vi "Save Data Functional Global.vi"(6 "Input Parameters":T1={"Points Per A-Scan"=0, "A-Scans per B-Scan"=0, "Voltage Range"=4.0, "Card Resolution (bits)"=16}, 7 "States":T2=enum."Initialize", 8 "error in (no error)":errorcluster, 9 "Folder":path, 10 "U16 Array":u16[](array[numeric]), 11 "Data Format":T3) -> (0 "error out":errorcluster, 3 "Saving Queue Out":refnum<queue>, 4 "# elements in queue":i32, 5 "Time Out":bool)   [LabVIEW 2014]
doc: "Functional global for saving OCT data. The data can either be 1 channel, 2 channel interleaved (ex. ATS 9462), or 2 channels appended (ATS 660). A state exists where the folder and files are created. Once this is complete, data can be enqueued to the VI."
uses:
  Type Defs/OCT DAQ Channel Data Type.ctl
  Saving Data States.ctl
  Type Defs/OCT Imaging Parameters Cluster.ctl
panel:
  out "Numeric":i32
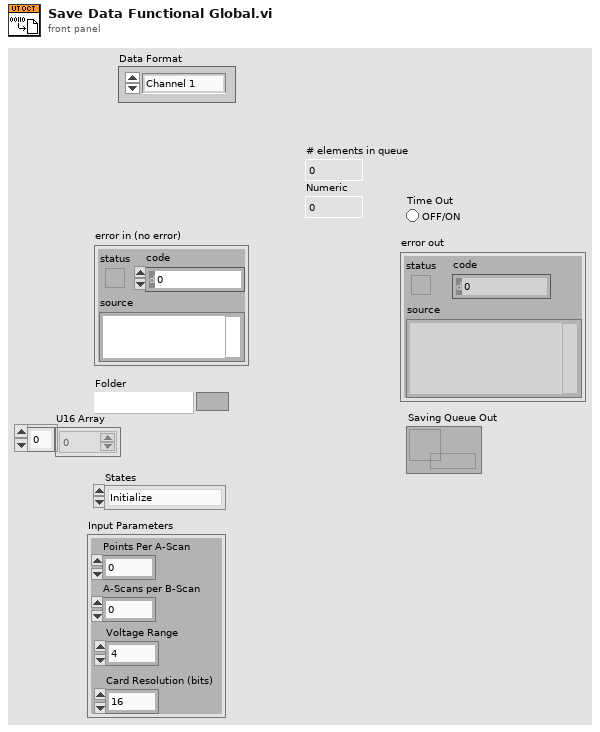
[diagram p1: front panel]
types:
  T1 = typedef "OCT Imaging Parameters Cluster.ctl" = cluster{"Points Per A-Scan":i32, "A-Scans per B-Scan":i32, "Voltage Range":sgl, "Card Resolution (bits)":u16}
  T2 = typedef "Saving Data States.ctl" = enum16{"Get Queue Size", "Get Queue", "Get Timeout", "Flush Queue", "Close Files", "Create Files", "Do Nothing", "Initialize", "Enqueue Data", "Save Data", "Shutdown"}
  T3 = typedef "OCT DAQ Channel Data Type.ctl" = enum16{"Channel 1", "Channel 2", "Channel 1 and 2"}
  T4 = enum16{"open", "replace", "create", "open or create", "replace or create", "replace or create with confirmation"}
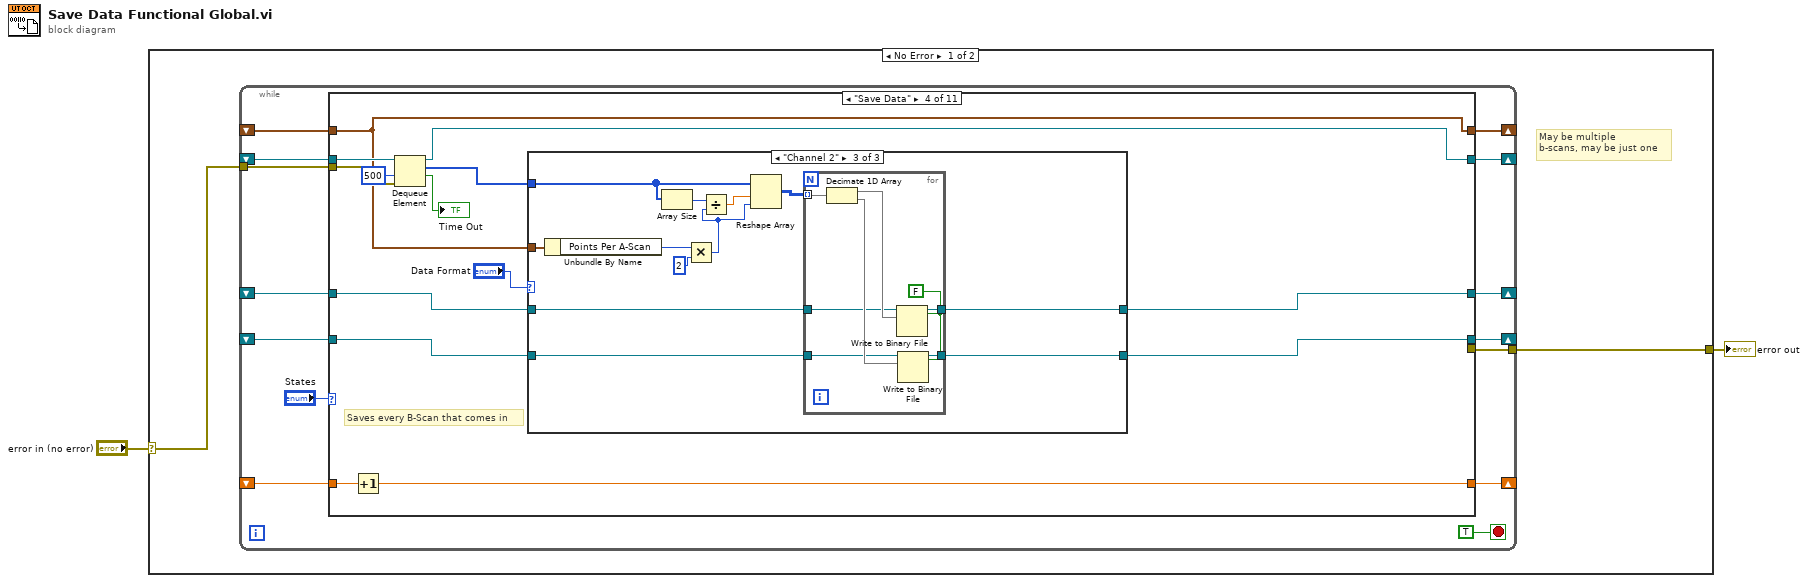
[diagram p0: block diagram]
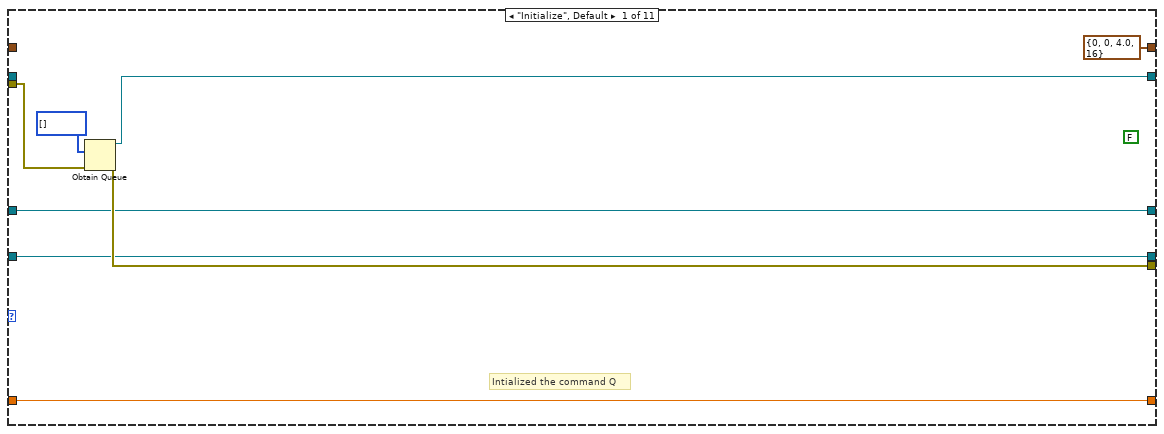
[diagram p2: hidden frame]
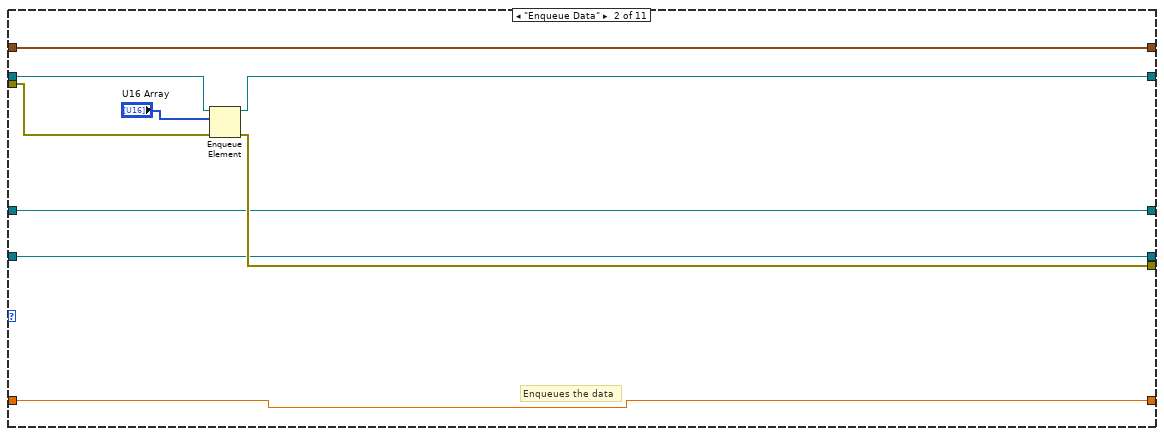
[diagram p3: hidden frame]
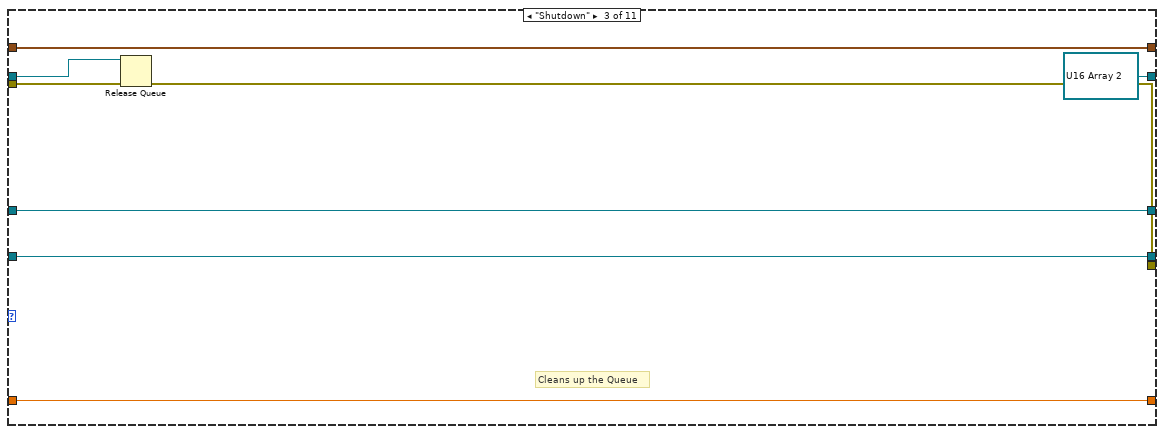
[diagram p4: hidden frame]
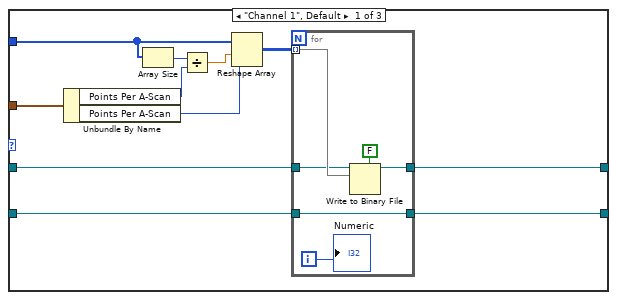
[diagram p5: hidden frame]
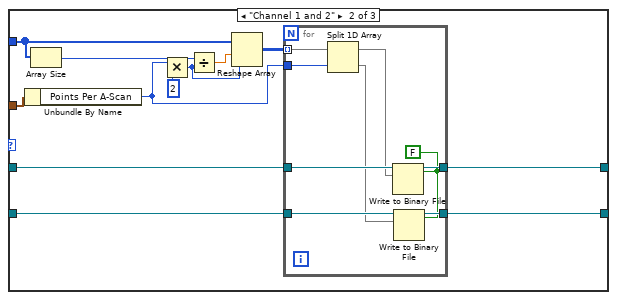
[diagram p6: hidden frame]
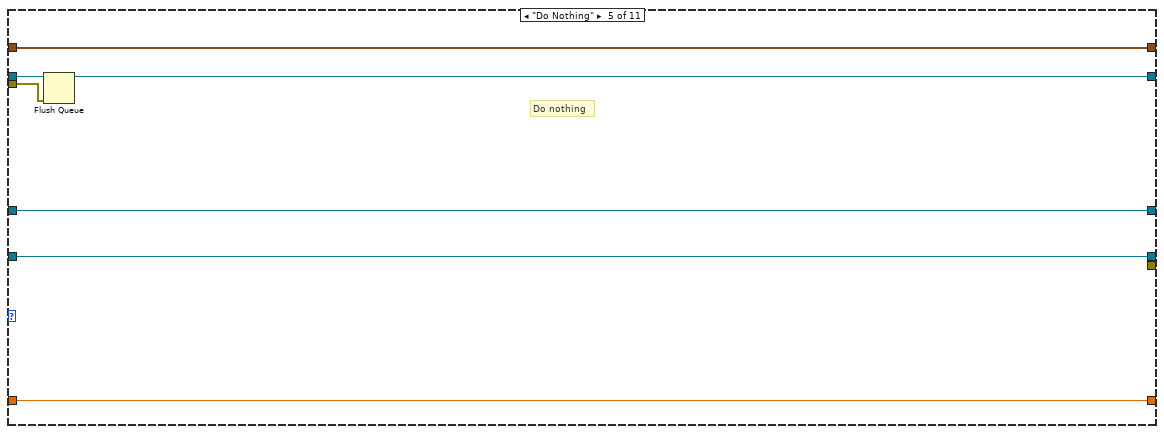
[diagram p7: hidden frame]
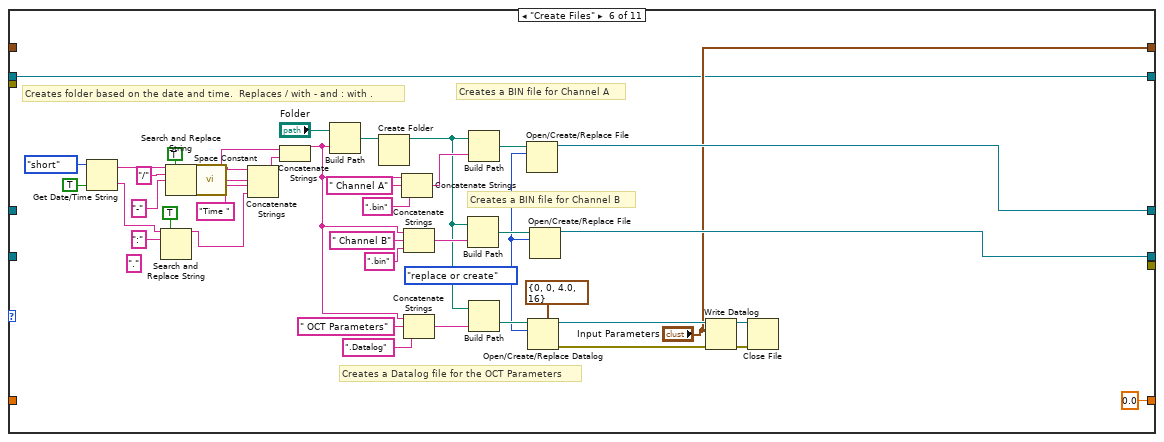
[diagram p8: hidden frame]
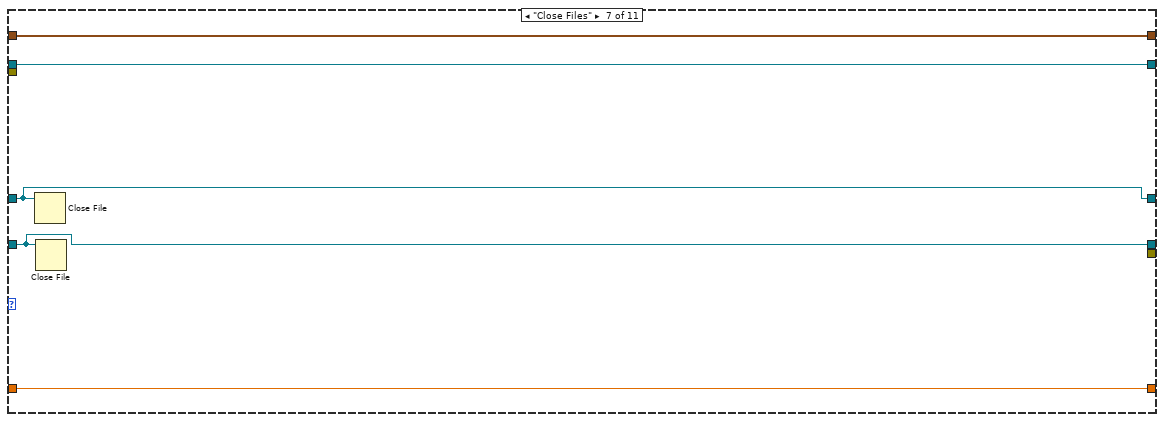
[diagram p9: hidden frame]
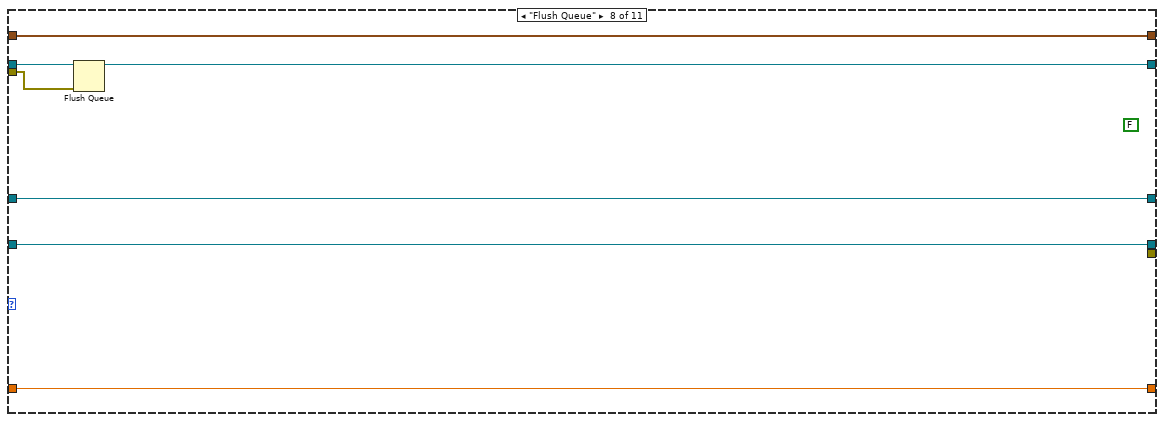
[diagram p10: hidden frame]
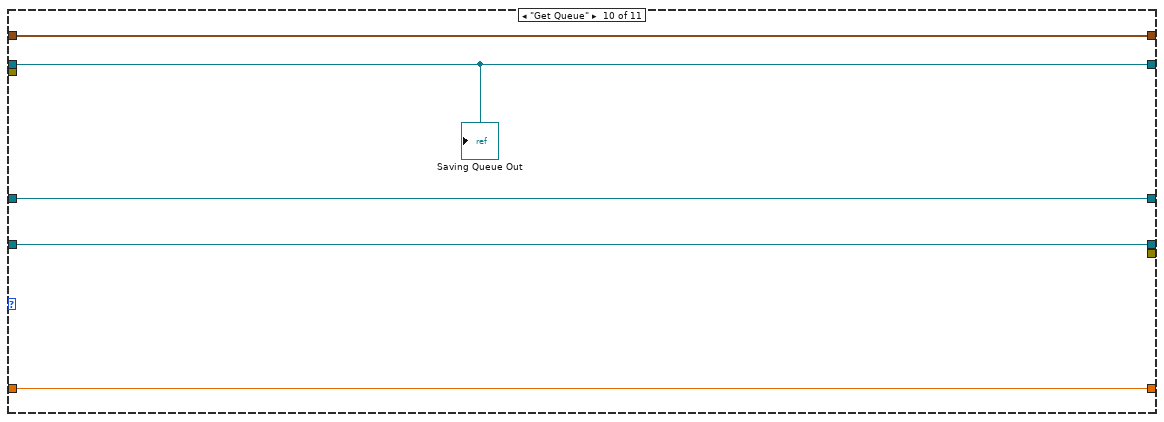
[diagram p12: hidden frame]
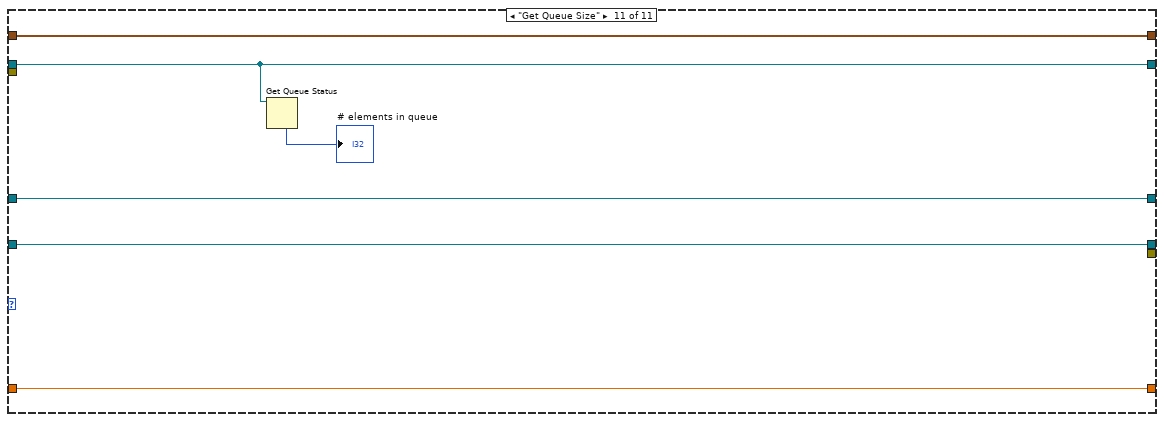
[diagram p13: hidden frame]
diagram:
  n1 = case shown="No Error" "error in (no error)" {
    selector: "error in (no error)" -> [w4 w192]
    tunnel: [w3 w192] -> w1
    frame No Error {
      # "May be multiple\nb-scans, may be just one"
      n2 = while {
        shift-right: [w12] -> _
        shift-left: _ -> [w16]
        tunnel: w4 -> [w17]
        tunnel: [w15] -> w3
        shift-right: [w14] -> _
        shift-left: _ -> [w13]
        shift-right: [w10] -> _
        shift-left: _ -> [w9]
        shift-right: [w8] -> _
        shift-left: _ -> [w7]
        shift-right: [w5] -> _
        shift-left: _ -> [w6]
        stop <- TRUE stop-if-true
        n3 = case shown="\"Save Data\"" "States" {
          tunnel: [w25 w34 refnum<queue> refnum ("queue out") w56 w117 w124 w165 w170 w177 w185 w188] -> w12
          tunnel: w17 -> [w26 w33 w41 w55 w118 _ _ w171 _ _ _]
          tunnel: w16 -> [_ w35 w43 w57 w119 w124 w165 w172 w177 w185 w188]
          tunnel: [w24 w32 w40 _ _ _ _ _ _ _ _] -> w15
          tunnel: [T1 {"Points Per A-Scan"=0, "A-Scans per B-Scan"=0, "Voltage Range"=4.0, "Card Resolution (bits)"=16} ("Input Parameters") w31 w42 w54 w122 "Input Parameters" w166 w173 w178 w184 w191] -> w14
          tunnel: w13 -> [_ w31 w42 w54 w122 _ w166 w173 w178 w184 w191]
          tunnel: [w22 w30 w39 w51 w121 w145 w167 w175 w180 w183 w190] -> w10
          tunnel: w9 -> [w22 w30 w39 w50 w121 _ w167 w175 w180 w183 w190]
          tunnel: [w21 w29 w38 w49 w120 w138 w168 w174 w179 w182 w189] -> w8
          tunnel: w7 -> [w21 w29 w38 w48 w120 _ w168 w174 w179 w182 w189]
          tunnel: w6 -> [w19 w27 w36 w45 w116 _ w164 w169 w176 w181 w186]
          tunnel: [w19 w27 w36 w44 w116 0.0 w164 w169 w176 w181 w186] -> w5
          frame "Initialize", Default {
            (unwired) FALSE ("timed out?")
            # "Intialized the command Q"
            n4 = Obtain Queue(element data type=u16[] [] ("U16 Array 2"), error in (no error)=w26) -> (queue out=w25:refnum<queue>, error out=w24:errorcluster)  [unwired: 3 in, 1 out]
          }
          frame "Enqueue Data" {
            # "Enqueues the data"
            n5 = Enqueue Element(queue=w35, element="U16 Array", error in (no error)=w33) -> (queue out=w34:refnum<queue>, error out=w32:errorcluster)  [unwired: 1 in, 1 out]
          }
          frame "Shutdown" {
            # "Cleans up the Queue"
            n6 = Release Queue(queue=w43, error in (no error)=w41) -> (error out=w40:errorcluster)  [unwired: 1 in, 2 out]
          }
          frame "Save Data" {
            # "Saves every B-Scan that comes in"
            n7 = Increment(x=w45) -> (x+1=w44:dbl)
            n8 = Dequeue Element(queue=w57, timeout in ms (-1)=500, error in (no error)=w55) -> (queue out=w56:refnum<queue>, element=w46:u16[], timed out?=→"Time Out":bool)  [unwired: 1 out]
            n9 = case shown="\"Channel 2\"" "Data Format" {
              tunnel: w46 -> [w65 w84 w105]
              tunnel: w54 -> [w66 w85 w106]
              tunnel: [w63 w81 w103] -> w51
              tunnel: w50 -> [w58 w78 w102]
              tunnel: w48 -> [w62 w79 w101]
              tunnel: [w61 w80 w100] -> w49
              frame "Channel 1", Default {
                n10 = Unbundle By Name(w66) -> ("Points Per A-Scan"=w68:i32, "Points Per A-Scan"=w59:i32)
                n11 = Array Size(array=w65) -> (size(s)=w67:i32)
                n12 = Divide(x=w67, y=w68) -> (x/y=w60:dbl)
                n13 = Reshape Array(w65, w60, w59) -> (w64:u16[][])
                n14 = for {
                  tunnel: w64 -> [w73] mode=indexing
                  tunnel: [w74] -> w63
                  tunnel: w62 -> [w71]
                  tunnel: [w71] -> w61
                  tunnel: w58 -> [w70]
                  i -> [w69]
                  n15 = Write to Binary File(file (use dialog)=w70, data=w73, 5:FALSE ("prepend array or string size? (T)")) -> (refnum out=w74:refnum<file>)  [unwired: 3 in, 2 out]
                  "Numeric" <- w69
                }
              }
              frame "Channel 1 and 2" {
                n16 = Unbundle By Name(w85) -> ("Points Per A-Scan"=w75:i32)
                n17 = Array Size(array=w84) -> (size(s)=w86:i32)
                n18 = Multiply(x=w75, y=2) -> (x*y=w76:i32)
                n19 = Divide(x=w86, y=w76) -> (x/y=w77:dbl)
                n20 = Reshape Array(w84, w77, w76) -> (w82:u16[][])
                n21 = for {
                  tunnel: w82 -> [w95] mode=indexing
                  tunnel: w75 -> [w94]
                  tunnel: [w93] -> w81
                  tunnel: [w92] -> w80
                  tunnel: w79 -> [w91]
                  tunnel: w78 -> [w90]
                  w87 = FALSE ("prepend array or string size? (T)")
                  n22 = Split 1D Array(array=w95, index=w94) -> (first subarray=w89:u16[], second subarray=w88:u16[])
                  n23 = Write to Binary File(file (use dialog)=w90, data=w89, 5:w87) -> (refnum out=w93:refnum<file>)  [unwired: 3 in, 2 out]
                  n24 = Write to Binary File(file (use dialog)=w91, data=w88, 5:w87) -> (refnum out=w92:refnum<file>)  [unwired: 3 in, 2 out]
                }
              }
              frame "Channel 2" {
                n25 = Unbundle By Name(w106) -> ("Points Per A-Scan"=w98:i32)
                n26 = Array Size(array=w105) -> (size(s)=w107:i32)
                n27 = Multiply(x=w98, y=2) -> (x*y=w96:i32)
                n28 = Divide(x=w107, y=w96) -> (x/y=w99:dbl)
                n29 = Reshape Array(w105, w99, w96) -> (w104:u16[][])
                n30 = for {
                  tunnel: w104 -> [w115] mode=indexing
                  tunnel: [w114] -> w103
                  tunnel: w102 -> [w111]
                  tunnel: w101 -> [w110]
                  tunnel: [w109] -> w100
                  w108 = FALSE ("prepend array or string size? (T)")
                  n31 = Decimate 1D Array(w115) -> (w113:u16[], w112:u16[])
                  n32 = Write to Binary File(file (use dialog)=w111, data=w113, 5:w108) -> (refnum out=w114:refnum<file>)  [unwired: 3 in, 2 out]
                  n33 = Write to Binary File(file (use dialog)=w110, data=w112, 5:w108) -> (refnum out=w109:refnum<file>)  [unwired: 3 in, 2 out]
                }
              }
            }
          }
          frame "Do Nothing" {
            # "Do nothing"
            n34 = Flush Queue(queue=w119, error in (no error)=w118) -> (queue out=w117:refnum<queue>)  [unwired: 2 out]
          }
          frame "Create Files" {
            w131 = T4."replace or create" ("operation (0:open)")
            (unwired) "." ("search string")
            # "Creates a Datalog file for the OCT Parameters"
            # "Creates a BIN file for Channel B"
            # "Creates a BIN file for Channel A"
            # "Creates folder based on the date and time.  Replaces / with - and : with ."
            n35 = Get Date/Time String(date format (0)=enum16{"short", "long", "abbreviated"}."short", want seconds? (F)=TRUE) -> (date string=w157:string, time string=w161:string)  [unwired: 1 in]
            n36 = Search and Replace String(replace all?=TRUE ("replace all? (F)"), input string=w161, search string=":") -> (result string=w151:string)  [unwired: 5 in, 3 out]
            n37 = Search and Replace String(replace all?=TRUE ("replace all? (F)"), input string=w157, search string="/", replace string="-" ("search string")) -> (result string=w153:string)  [unwired: 4 in, 3 out]
            n38 = call <vilib>:"Space Constant.vi"() -> ("String"=w160:string)
            n39 = Concatenate Strings(w153, w160, "Time " ("search string"), w151) -> (w159:string)
            n40 = Concatenate Strings(w160, w159) -> (w135:string)
            n41 = Build Path(base path="Folder", name or relative path=w135) -> (appended path=w148:path)
            n42 = Create Folder(path (use dialog)=w148) -> (created path=w132:path)  [unwired: 2 in, 2 out]
            n43 = Concatenate Strings(w135, " Channel A" ("string"), ".bin" ("search string")) -> (w147:string)
            n44 = Concatenate Strings(w135, " Channel B" ("string"), ".bin" ("search string")) -> (w140:string)
            n45 = Concatenate Strings(w135, " OCT Parameters" ("string"), ".Datalog" ("search string")) -> (w133:string)
            n46 = Build Path(base path=w132, name or relative path=w140) -> (appended path=w139:path)
            n47 = Build Path(base path=w132, name or relative path=w147) -> (appended path=w146:path)
            n48 = Build Path(base path=w132, name or relative path=w133) -> (appended path=w134:path)
            n49 = Open/Create/Replace File(file path (use dialog)=w146, operation (0:open)=w131) -> (refnum out=w145:refnum<file>)  [unwired: 4 in, 2 out]
            n50 = Open/Create/Replace Datalog(5:T1 {"Points Per A-Scan"=0, "A-Scans per B-Scan"=0, "Voltage Range"=4.0, "Card Resolution (bits)"=16} ("Input Parameters"), 10:w131, 11:w134) -> (0:w128:errorcluster, 3:w129:refnum<k1>)  [unwired: 3 in, 1 out]
            n51 = Open/Create/Replace File(file path (use dialog)=w139, operation (0:open)=w131) -> (refnum out=w138:refnum<file>)  [unwired: 4 in, 2 out]
            n52 = Write Datalog(4:w128, 6:"Input Parameters", 7:w129) -> (0:w127:errorcluster, 3:w126:refnum<k1>)
            n53 = Close File(refnum=w126, error in=w127) -> ()  [unwired: 2 out]
          }
          frame "Close Files" {
            n54 = Close File(refnum=w167) -> ()  [unwired: 1 in, 2 out]
            n55 = Close File(refnum=w168) -> ()  [unwired: 1 in, 2 out]
          }
          frame "Flush Queue" {
            (unwired) FALSE ("timed out?")
            n56 = Flush Queue(queue=w172, error in (no error)=w171) -> (queue out=w170:refnum<queue>)  [unwired: 2 out]
          }
          frame "Get Timeout" {
          }
          frame "Get Queue" {
            "Saving Queue Out" <- w185
          }
          frame "Get Queue Size" {
            n57 = Get Queue Status(queue=w188) -> (# elements in queue=→"# elements in queue":i32)  [unwired: 2 in, 7 out]
          }
        }
      }
    }
    frame Error {
    }
  }
  "error out" <- w1
